vi "Read_Serial_Port_Emulator_Test.vi"() -> ()   [LabVIEW 2017]
uses:
  Classes/ADCP.lvclass
panel:
  in  "ADCP in":refnum<class "ADCP.lvclass">
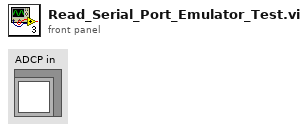
[diagram p1: front panel]
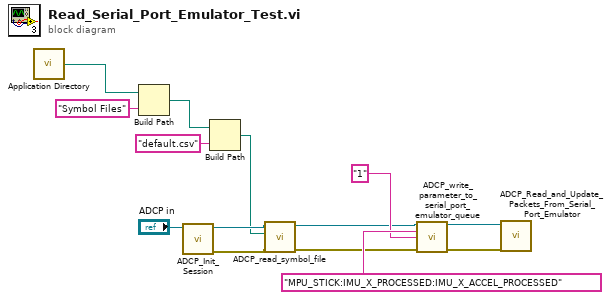
[diagram p0: block diagram]
diagram:
  n1 = call <vilib>:"Application Directory.vi"() -> ("Application Directory"=w6:path)
  n2 = Build Path(base path=w6, name or relative path="Symbol Files") -> (appended path=w4:path)
  n3 = call "ADCP_Init_Session.vi"("ADCP in"="ADCP in") -> ("error out"=w9:errorcluster, "ADCP out"=w10:refnum<class "ADCP.lvclass">)  [unwired: 9 in]
  n4 = Build Path(base path=w4, name or relative path="default.csv") -> (appended path=w2:path)
  n5 = call "ADCP_read_symbol_file.vi"("error in (no error)"=w9, "Symbol File Path"=w2, "ADCP in"=w10) -> ("error out"=w8:errorcluster, "ADCP out"=w7:refnum<class "ADCP.lvclass">)  [unwired: 5 in, 2 out]
  n6 = call "ADCP_write_parameter_to_serial_port_emulator_queue.vi"("ADCP In"=w7, "Parameter Name"="MPU_STICK:IMU_X_PROCESSED:IMU_X_ACCEL_PROCESSED", "Parameter Value"="1", "error in (no error)"=w8) -> ("ADCP out"=w12:refnum<class "ADCP.lvclass">, "error out"=w11:errorcluster)  [unwired: 10 in]
  n7 = call "ADCP_Read_and_Update_Packets_From_Serial_Port_Emulator.vi"("error in (no error)"=w11, "ADCP In"=w12) -> ()  [unwired: 6 in, 4 out]
